vi "Module Type.vi"(11 "Telemetry Server in":refnum<class "Telemetry Server.lvclass">) -> (2 "Module Type":string)   [LabVIEW 2020, in "VolatusTelemetry.lvlib" / "Telemetry Server.lvclass"]
uses:
  Telemetry Server.lvclass
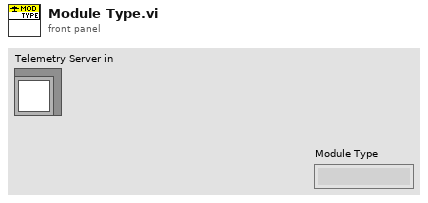
[diagram p1: front panel]
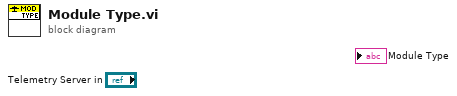
[diagram p0: block diagram]
diagram:
